vi "get_hard_limit_option_by_name.vi"(8 "error in (no error)":errorcluster caption="错误输入（无错误）", 10 "name":string, 11 "MotorSystem输入":refnum<class "MotorSystem.lvclass">) -> (0 "error out":errorcluster caption="错误输出", 2 "hard limit option":T1, 3 "MotorSystem输出":refnum<class "MotorSystem.lvclass">)   [LabVIEW 2016, in "MotionControl_UFO_3DOF.lvlib" / "MotorSystem.lvclass"]
uses:
  <userlib>/MotionControl_UFO_3DOF/MotorSystem/MotorSystem.lvclass
  <userlib>/MotionControl_UFO_3DOF/OneMotion/hard limit option.ctl
  <userlib>/MotionControl_UFO_3DOF/MotorSystem/MotorSystem.lvclass/MotorSystem.ctl
  <userlib>/MotionControl_UFO_3DOF/OneMotion/OneMotion.lvclass
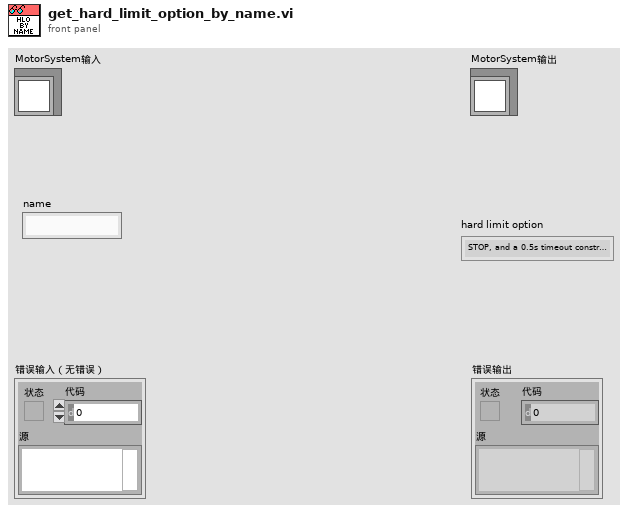
[diagram p1: front panel]
types:
  T1 = typedef "MotionControl_UFO_3DOF.lvlib/OneMotion.lvclass/hard limit option.ctl" = enum16{"STOP, and a 0.5s timeout constraint in move", "STOP, and move disabled"}
  T2 = typedef "MotionControl_UFO_3DOF.lvlib/MotorSystem.lvclass/MotionCluster.ctl" = cluster{"OneMotion.lvclass":refnum<class "OneMotion.lvclass">, "connected?":bool, "default enabled?":bool, "enabled?":bool}
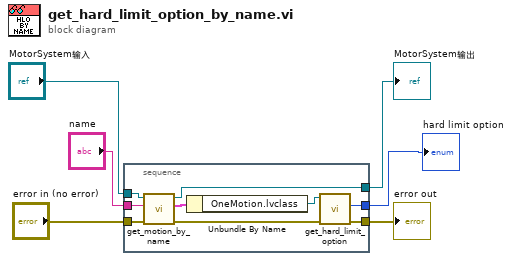
[diagram p0: block diagram]
diagram:
  n1 = stacked-sequence {
    tunnel: [w7] -> w6
    tunnel: [w11] -> w4
    tunnel: "MotorSystem输入" -> [w15]
    tunnel: "name" -> [w14]
    tunnel: [w10] -> w1
    tunnel: "error in (no error)" -> [w9]
    frame #0 {
      n2 = call <userlib>:"get_motion_by_name.vi"("error in (no error)"=w9, "name"=w14, "MotorSystem in"=w15) -> ("error out"=w8:errorcluster, "motion cluster"=w13:T2, "MotorSystem out"=w11:refnum<class "MotorSystem.lvclass">)  [unwired: 6 in]
      n3 = Unbundle By Name(w13) -> ("OneMotion.lvclass"=w12:refnum<class "OneMotion.lvclass">)
      n4 = call-dynamic "get_hard_limit_option.vi"("error in (no error)"=w8, "OneMotion输入"=w12) -> ("error out"=w7:errorcluster, "hard limit option"=w10:T1)  [unwired: 7 in, 1 out]
    }
  }
  "error out" <- w6
  "MotorSystem输出" <- w4
  "hard limit option" <- w1
